vi "Check parts acceptable - toplayer.vi"(6 "Stack IDs":string[](array[string]), 7 "DB out stack":string[][](array[string]), 8 "error in (no error)":errorcluster, 9 "Toplayer IDs":string[](array[string]), 10 "DB out top":string[][](array[string]), 11 "Database Entry in":refnum<class "Database Entry.lvclass">) -> (0 "error out":errorcluster, 2 "Replace parts out":bool, 3 "Database Entry out":refnum<class "Database Entry.lvclass">, 4 "Abort?":bool)   [LabVIEW 2021, in "Database Entry.lvclass"]
uses:
  Database Entry.lvclass
panel:
  in  "Database out - stack":i32[](listbox)
  in  "Replace parts top":bool
  in  "Are these parts satisfactory?":bool
  in  "Abort":bool
  in  "Submit":bool
  in  "Database out - toplayer":i32[](listbox)
  # "(If parts are satisfactory, this assembly run will be written into Postgres.)"
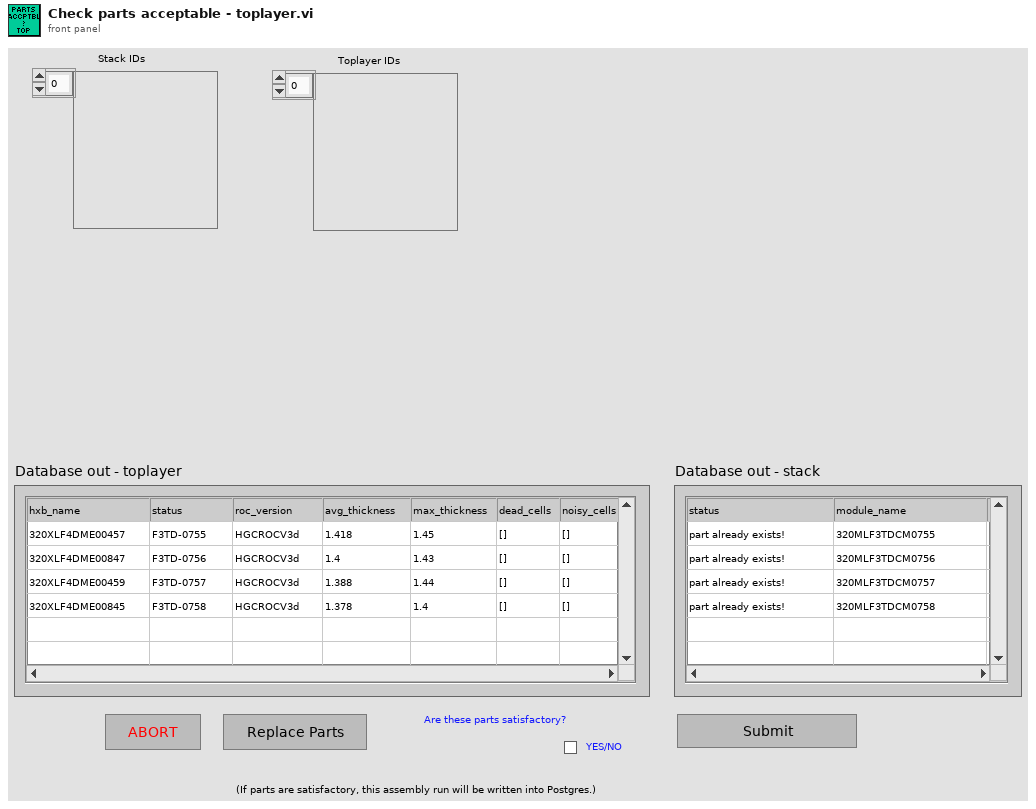
[diagram p1: front panel]
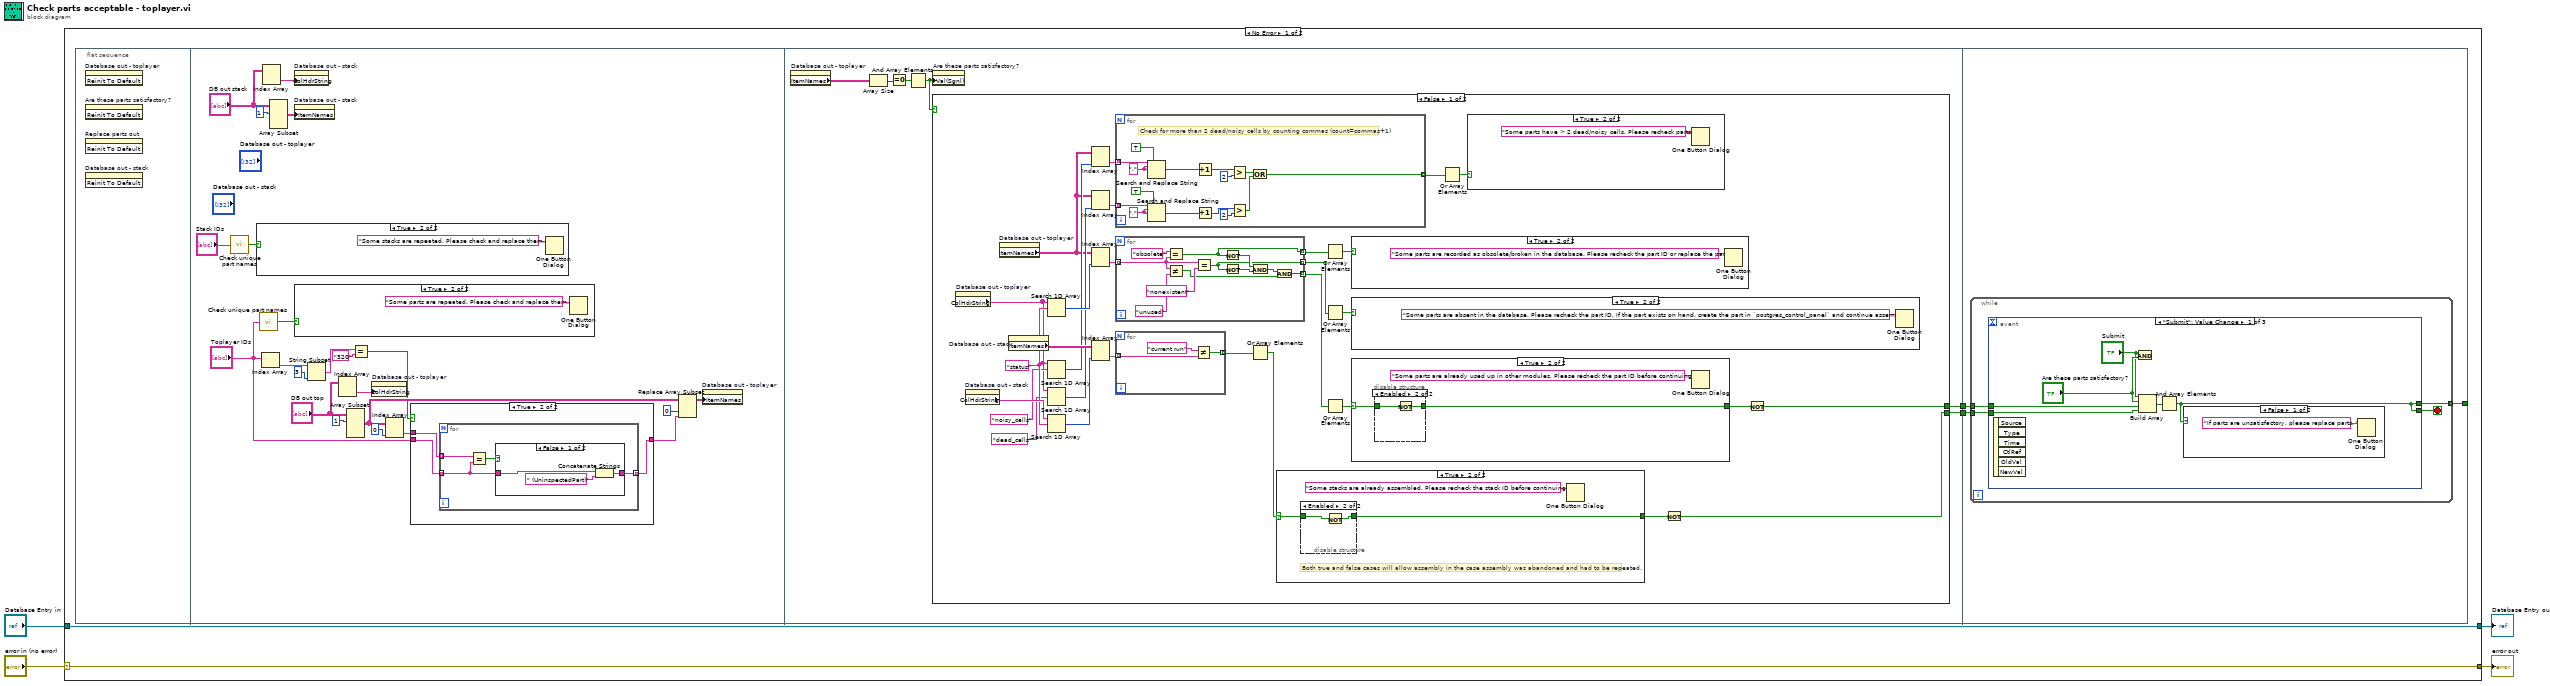
[diagram p0: block diagram]
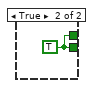
[diagram p13: hidden frame]
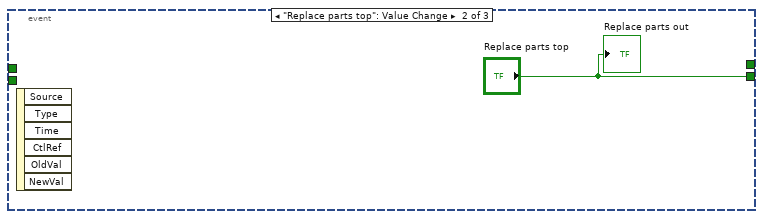
[diagram p15: hidden frame]
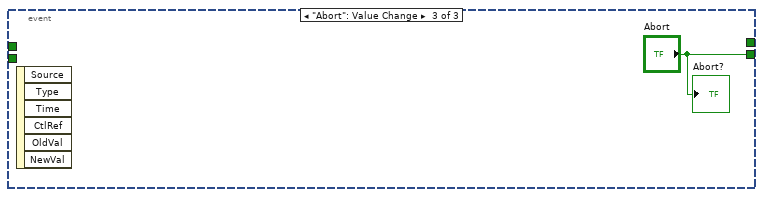
[diagram p16: hidden frame]
diagram:
  n1 = case shown="No Error" "error in (no error)" {
    selector: "error in (no error)" -> [w8 w144]
    tunnel: [w8 w144] -> w3
    tunnel: [w7 w143] -> w1
    tunnel: "Database Entry in" -> [w7 w143]
    frame No Error {
      n2 = flat-sequence {
        tunnel: [w46] -> w6
        tunnel: [w45] -> w5
        tunnel: [w129] -> _
        tunnel: w6 -> [w128]
        tunnel: w5 -> [w127]
        frame #0 {
          n3 = invoke on="Database out - toplayer" class="MCListbox (strict)" method="Reinit To Default"() -> ()  [unwired: 3 in, 3 out]
          n4 = invoke on="Are these parts satisfactory?" class="Bool (strict)" method="Reinit To Default"() -> ()  [unwired: 3 in, 3 out]
          n5 = invoke on="Replace parts out" class="Bool (strict)" method="Reinit To Default"() -> ()  [unwired: 3 in, 3 out]
          n6 = invoke on="Database out - stack" class="MCListbox (strict)" method="Reinit To Default"() -> ()  [unwired: 3 in, 3 out]
        }
        frame #1 {
          n7 = call "Check unique part names.vi"("Part IDs"="Stack IDs") -> ("Parts repeated"=w13:bool)
          n8 = case shown="True" w13 {
            frame False {
            }
            frame True {
              n9 = One Button Dialog(message="Some stacks are repeated. Please check and replace them.") -> ()  [unwired: 1 in, 1 out]
            }
          }
          n10 = call "Check unique part names.vi"("Part IDs"="Toplayer IDs") -> ("Parts repeated"=w15:bool)
          n11 = Index Array(array="Toplayer IDs") -> (element=w21:string)  [unwired: 1 in]
          n12 = Index Array(array="DB out stack") -> (element=w12:string[])  [unwired: 2 in]
          n13 = Array Subset(array="DB out stack", index (row)=1 ("index")) -> (w10:string[][])  [unwired: 3 in]
          n14 = property on="Database out - stack" class="MCListbox (strict)"("ColHdrString"=w12) -> ()  [unwired: 2 in, 2 out]
          n15 = property on="Database out - stack" class="MCListbox (strict)"("ItemNames"=w10) -> ()  [unwired: 2 in, 2 out]
          n16 = case shown="True" w15 {
            frame False {
            }
            frame True {
              n17 = One Button Dialog(message="Some parts are repeated. Please check and replace them.") -> ()  [unwired: 1 in, 1 out]
            }
          }
          n18 = String Subset(string=w21, length (rest)=3 ("length (rest)")) -> (substring=w17:string)  [unwired: 1 in]
          n19 = Index Array(array="DB out top") -> (element=w23:string[])  [unwired: 2 in]
          n20 = Array Subset(array="DB out top", index (row)=1 ("index")) -> (w27:string[][])  [unwired: 3 in]
          n21 = Equal?(x=w17, y="320") -> (x = y?=w19:bool)
          n22 = property on="Database out - toplayer" class="MCListbox (strict)"("ColHdrString"=w23) -> ()  [unwired: 2 in, 2 out]
          n23 = Index Array(array=w27, index (col)=0 ("disabled index (col)")) -> (element=w28:string[])  [unwired: 1 in]
          n24 = case shown="True" w19 {
            tunnel: w28 -> [_ w36]
            tunnel: [w33 w35] -> w25
            tunnel: "Toplayer IDs" -> [w33 w34]
            frame False {
            }
            frame True {
              n25 = for {
                tunnel: w36 -> [w39] mode=indexing
                tunnel: w34 -> [w37] mode=indexing
                tunnel: [w38] -> w35 mode=indexing
                n26 = Equal?(x=w39, y=w37) -> (x = y?=w40:bool)
                n27 = case shown="False" w40 {
                  tunnel: w37 -> [w43 w44]
                  tunnel: [w41 w44] -> w38
                  frame False {
                    n28 = Concatenate Strings(w43, " (UninspectedPart)" ("string")) -> (w41:string)
                  }
                  frame True {
                  }
                }
              }
            }
          }
          n29 = Replace Array Subset(array=w27, new element=w25, index (col)=0 ("disabled index (col)")) -> (w22:string[][])  [unwired: 1 in]
          n30 = property on="Database out - toplayer" class="MCListbox (strict)"("ItemNames"=w22) -> ()  [unwired: 2 in, 2 out]
        }
        frame #2 {
          n31 = property on="Database out - toplayer" class="MCListbox (strict)"() -> ("ItemNames"=w48:string[][])  [unwired: 2 in, 2 out]
          n32 = Array Size(array=w48) -> (size(s)=w49:i32[])
          n33 = Equal To 0?(x=w49) -> (x = 0?=w50:bool[])
          n34 = And Array Elements(Boolean array=w50) -> (logical AND=w47:bool)
          n35 = property on="Are these parts satisfactory?" class="Bool (strict)"("Val(Sgnl)"=w47) -> ()  [unwired: 2 in, 2 out]
          n36 = case shown="False" w47 {
            tunnel: [w69 w126] -> w46
            tunnel: [w67 w126] -> w45
            frame False {
              w74 = "status" ("element")
              n37 = property on="Database out - toplayer" class="MCListbox (strict)"() -> ("ColHdrString"=w56:string[])  [unwired: 2 in, 2 out]
              n38 = property on="Database out - stack" class="MCListbox (strict)"() -> ("ColHdrString"=w75:string[])  [unwired: 2 in, 2 out]
              n39 = property on="Database out - toplayer" class="MCListbox (strict)"() -> ("ItemNames"=w54:string[][])  [unwired: 2 in, 2 out]
              n40 = property on="Database out - stack" class="MCListbox (strict)"() -> ("ItemNames"=w73:string[][])  [unwired: 2 in, 2 out]
              n41 = Search 1D Array(1D array=w56, element=w74) -> (index of element=w65:i32)  [unwired: 1 in]
              n42 = Search 1D Array(1D array=w56, element="noisy_cells") -> (index of element=w55:i32)  [unwired: 1 in]
              n43 = Search 1D Array(1D array=w56, element="dead_cells") -> (index of element=w59:i32)  [unwired: 1 in]
              n44 = Search 1D Array(1D array=w75, element=w74) -> (index of element=w63:i32)  [unwired: 1 in]
              n45 = Index Array(array=w54, index (col)=w55) -> (element=w53:string[])  [unwired: 1 in]
              n46 = Index Array(array=w54, index (col)=w59) -> (element=w58:string[])  [unwired: 1 in]
              n47 = Index Array(array=w54, index (col)=w65) -> (element=w66:string[])  [unwired: 1 in]
              n48 = Index Array(array=w73, index (col)=w63) -> (element=w64:string[])  [unwired: 1 in]
              n49 = for {
                tunnel: w58 -> [w94] mode=indexing
                tunnel: w53 -> [w84] mode=indexing
                tunnel: [w81] -> w52 mode=indexing
                w88 = "," ("search string")
                w93 = "," ("search string")
                # "Check for more than 2 dead/noisy cells by counting commas (count=commas+1)"
                n50 = Search and Replace String(replace all?=TRUE ("replace all? (F)"), input string=w84, search string=w88, replace string=w88) -> (number of replacements=w87:i32)  [unwired: 4 in, 3 out]
                n51 = Search and Replace String(replace all?=TRUE ("replace all? (F)"), input string=w94, search string=w93, replace string=w93) -> (number of replacements=w92:i32)  [unwired: 4 in, 3 out]
                n52 = Increment(x=w87) -> (x+1=w86:i32)
                n53 = Increment(x=w92) -> (x+1=w91:i32)
                n54 = Greater?(x=w86, y=2) -> (0:w83:bool)
                n55 = Greater?(x=w91, y=2) -> (0:w82:bool)
                n56 = Or(x=w83, y=w82) -> (x .or. y?=w81:bool)
              }
              n57 = for {
                tunnel: w66 -> [w120] mode=indexing
                tunnel: [w122] -> w79 mode=indexing
                tunnel: [w116] -> w78 mode=indexing
                tunnel: [w117] -> w62 mode=indexing
                n58 = Equal?(x="obsolete" ("y"), y=w120) -> (x = y?=w117:bool)
                n59 = Not Equal?(x=w120, y="unused") -> (x != y?=w123:bool)
                n60 = Equal?(x=w120, y="nonexistent") -> (x = y?=w116:bool)
                n61 = Not(x=w117) -> (.not. x?=w119:bool)
                n62 = Not(x=w116) -> (.not. x?=w118:bool)
                n63 = And(x=w119, y=w118) -> (x .and. y?=w115:bool)
                n64 = And(x=w115, y=w123) -> (x .and. y?=w122:bool)
              }
              n65 = for {
                tunnel: w64 -> [w106] mode=indexing
                tunnel: [w105] -> w72 mode=indexing
                n66 = Not Equal?(x="current run" ("y"), y=w106) -> (x != y?=w105:bool)
              }
              n67 = Or Array Elements(Boolean array=w72) -> (logical OR=w71:bool)
              n68 = case shown="True" w71 {
                selector: w71 -> [w97 w99]
                tunnel: [w97 w98] -> w68
                frame False {
                }
                frame True {
                  # "Both true and false cases will allow assembly in the case assembly was abandoned and had to be repeated."
                  n69 = disable-structure shown="Enabled" {
                    disable-tunnel: w99 -> [w101 w103]
                    disable-tunnel: [w101 w102] -> w98
                    frame Disabled {
                    }
                    frame Enabled {
                      n70 = Not(x=w103) -> (.not. x?=w102:bool)
                    }
                  }
                  n71 = One Button Dialog(message="Some stacks are already assembled. Please recheck the stack ID before continuing.") -> ()  [unwired: 1 in, 1 out]
                }
              }
              n72 = Or Array Elements(Boolean array=w62) -> (logical OR=w61:bool)
              n73 = Or Array Elements(Boolean array=w78) -> (logical OR=w77:bool)
              n74 = Or Array Elements(Boolean array=w79) -> (logical OR=w76:bool)
              n75 = case shown="True" w61 {
                frame False {
                }
                frame True {
                  n76 = One Button Dialog(message="Some parts are recorded as obsolete/broken in the database. Please recheck the part ID or replace the part.") -> ()  [unwired: 1 in, 1 out]
                }
              }
              n77 = case shown="True" w77 {
                frame False {
                }
                frame True {
                  n78 = One Button Dialog(message="Some parts are absent in the database. Please recheck the part ID. If the part exists on hand, create the part in `postgres_control_panel` and continue assembly. ") -> ()  [unwired: 1 in, 1 out]
                }
              }
              n79 = case shown="True" w76 {
                selector: w76 -> [w107 w109]
                tunnel: [w107 w108] -> w70
                frame False {
                }
                frame True {
                  n80 = disable-structure shown="Enabled" {
                    disable-tunnel: w109 -> [w111 w113]
                    disable-tunnel: [w111 w112] -> w108
                    frame Disabled {
                    }
                    frame Enabled {
                      n81 = Not(x=w113) -> (.not. x?=w112:bool)
                    }
                  }
                  n82 = One Button Dialog(message="Some parts are already used up in other modules. Please recheck the part ID before continuing.") -> ()  [unwired: 1 in, 1 out]
                }
              }
              n83 = Or Array Elements(Boolean array=w52) -> (logical OR=w51:bool)
              n84 = case shown="True" w51 {
                frame False {
                }
                frame True {
                  n85 = One Button Dialog(message="Some parts have > 2 dead/noisy cells. Please recheck parts.") -> ()  [unwired: 1 in, 1 out]
                }
              }
              n86 = Not(x=w68) -> (.not. x?=w67:bool)
              n87 = Not(x=w70) -> (.not. x?=w69:bool)
            }
            frame True {
              w126 = TRUE
            }
          }
        }
        frame #3 {
          n88 = while {
            tunnel: [w132] -> w129
            tunnel: w128 -> [w131]
            tunnel: w127 -> [w130]
            stop <- w133 stop-if-true
            n89 = event shown="[0] \"Submit\": Value Change" {
              selector: _ -> [_ _ _]
              dyn-events: _ -> [_ _ _]
              timeout: _ -> [_ _ _]
              tunnel: [w134 "Replace parts top" "Abort"] -> w133
              tunnel: [w134 _ _] -> w132
              tunnel: w131 -> [w137 _ _]
              tunnel: w130 -> [w136 _ _]
              event "Submit": Value Change {
                n90 = event-data() -> ()  [unwired: 1 in, 6 out]
                n91 = And(x="Submit", y="Are these parts satisfactory?") -> ()  [unwired: 1 out]
                n92 = Build Array("Submit", "Are these parts satisfactory?", w137, w136) -> (w135:bool[])
                n93 = And Array Elements(Boolean array=w135) -> (logical AND=w134:bool)
                n94 = case shown="False" w134 {
                  frame False {
                    n95 = One Button Dialog(message="If parts are unsatisfactory, please replace parts. ") -> ()  [unwired: 1 in, 1 out]
                  }
                  frame True {
                  }
                }
              }
              event "Replace parts top": Value Change {
                n96 = event-data() -> ()  [unwired: 1 in, 6 out]
                "Replace parts out" <- "Replace parts top"
              }
              event "Abort": Value Change {
                n97 = event-data() -> ()  [unwired: 1 in, 6 out]
                "Abort?" <- "Abort"
              }
            }
          }
        }
      }
    }
    frame Error {
    }
  }
  "error out" <- w3
  "Database Entry out" <- w1
